vi "Start_Vi.vi"(1 "VI-Pfad":path=path "E:/CryoTUM-Software/16T-Magnet_Ultimate-Control_Version_2-0/LS370Monitor.vi") -> ()   [LabVIEW 2018]
panel:
  out "LS 370 Monitor":T1(ring)
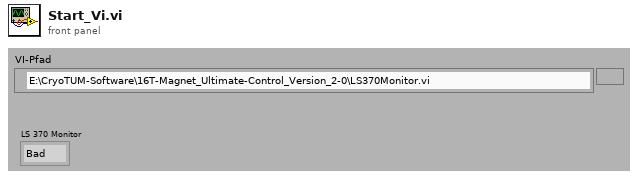
[diagram p1: front panel]
types:
  T1 = enum32{"Bad", "Idle", "Run top level", "Running"}
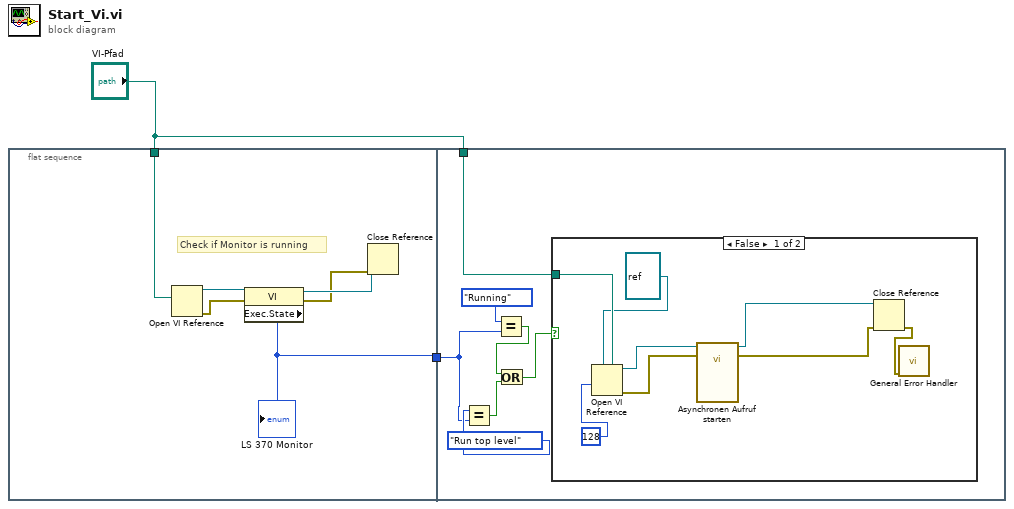
[diagram p0: block diagram]
diagram:
  n1 = flat-sequence {
    tunnel: [w5] -> w2
    tunnel: "VI-Pfad" -> [w3]
    tunnel: w2 -> [w12]
    tunnel: "VI-Pfad" -> [w9]
    frame #0 {
      # "Check if Monitor is running"
      n2 = Open VI Reference(vi path=w3) -> (vi reference=w4:refnum<vi>, error out=w8:errorcluster)  [unwired: 5 in]
      n3 = property class="VI"(reference=w4, error in=w8) -> (reference out=w7:refnum<vi>, error out=w6:errorcluster, "Exec.State"=w5:T1)
      "LS 370 Monitor" <- w5
      n4 = Close Reference(reference=w7, error in (no error)=w6) -> ()  [unwired: 1 out]
    }
    frame #1 {
      n5 = Equal?(x=T1."Run top level" ("LS 370 Monitor 2"), y=w12) -> (x = y?=w11:bool)
      n6 = Equal?(x=T1."Running" ("LS 370 Monitor 2"), y=w12) -> (x = y?=w14:bool)
      n7 = Or(x=w14, y=w11) -> (x .or. y?=w10:bool)
      n8 = case shown="False" w10 {
        tunnel: w9 -> [w23 _]
        frame False {
          n9 = Open VI Reference ("VI-Referenz öffnen")(type specifier VI Refnum (for type only)=refnum<vi> refnum ("vi reference"), vi path=w23, options=128) -> (vi reference=w22:refnum<vi>, error out=w21:errorcluster)  [unwired: 3 in]
          n10 = call-by-ref "Asynchronen Aufruf starten"(reference=w22, error in=w21) -> (reference out=w20:refnum<vi>, error out=w19:errorcluster)  [unwired: 1 in]
          n11 = Close Reference(reference=w20, error in (no error)=w19) -> (error out=w18:errorcluster)
          n12 = call <vilib>:"General Error Handler.vi"("error in (no error)"=w18) -> ()  [unwired: 10 in, 5 out]
        }
        frame True {
        }
      }
    }
  }
